vi "Autonomous Independent.vi"   [LabVIEW 2015]
doc: "This VI is called when autonomous begins, and will automatically be terminated when autonomous ends. You can carry out timed or sensor driven robot movement independently without needing to return to the caller."
uses:
  <vilib>/Rock Robotics/WPI/Solenoid/WPI_SolenoidValue.ctl
  <vilib>/Rock Robotics/WPI/Utilities/WPI_GetSetVariantRefNum.vi
  <vilib>/Rock Robotics/Network Tables/NT Read String.vi
  <vilib>/Rock Robotics/WPI/Solenoid/WPI_SolenoidSetEnum.vi
panel:
  # "Be sure to right-click and choose Data Operations>>Make Current Value default if you want to save the array values with the VI"
types:
  T1 = typedef "WPI_RobotDriveDevRef.ctl" = cluster{"DevStatus":errorcluster, "Motors[]":T2[], "Square Inputs":bool, "Max Output":dbl}
  T2 = typedef "WPI_MotorControlDeviceRef.ctl" = cluster{"DeviceStatus":errorcluster, "Type":T3, "PWM":cluster{"PWM Channel":T4, "DeadBand":T5}, "CAN":cluster{"Device Number":u8, "Control Mode":T6, "Semaphore":T7, "Max Vout":dbl, "TalonSRX Control Mode":T8}, "Invert":bool}
  T3 = typedef "WPI_MotorControlType.ctl" = enum16{"PWM", "CAN", "CANTalonSRX"}
  T4 = typedef "FPGA_DIOPWMChannel.ctl" = enum8{"PWM 0", "PWM 1", "PWM 2", "PWM 3", "PWM 4", "PWM 5", "PWM 6", "PWM 7", "PWM 8", "PWM 9", "PWM MXP 0", "PWM MXP 1", "PWM MXP 2", "PWM MXP 3", "PWM MXP 4", "PWM MXP 5", "PWM MXP 6", "PWM MXP 7", "PWM MXP 8", "PWM MXP 9", "Invalid"}
  T5 = typedef "WPI_PWMDeadband.ctl" = cluster{"Name":string, "maxPositivePwm":i32, "minPositivePwm":i32, "centerPwm":i32, "maxNegativePwm":i32, "minNegativePwm":i32, "angularRange":u16}
  T6 = typedef "WPI_CANJaguar_ControlMode.ctl" = enum8{"Percent VBus", "Current", "Speed", "Position", "Voltage"}
  T7 = typedef "Semaphore RefNum" = refnum<k1>
  T8 = typedef "WPI_CANTalonSRX_APIControlMode.ctl" = enum8{"Percent VBus", "Speed", "Position", "Slave", "Unchanged / Invalid", "Voltage Compensation", "Current", "Motion Profile"}
  T9 = typedef "WPI_SolenoidValue.ctl" = enum16{"Off", "On", "Forward", "Reverse"}
  T10 = typedef "WPI_SolenoidDevRef.ctl" = cluster{"DevStatus":errorcluster, "Pneumatics Control Module":u8, "Forward Solenoid Channel":T11, "Reverse Solenoid Channel":T11}
  T11 = typedef "WPI_SolenoidChannel.ctl" = enum8{"Solenoid 0", "Solenoid 1", "Solenoid 2", "Solenoid 3", "Solenoid 4", "Solenoid 5", "Solenoid 6", "Solenoid 7", "Invalid"}
  T12 = typedef "WPI_AccelerometerDevRef.ctl" = cluster{"DevStatus":errorcluster, "Scaling":T13, "Analog Channels":T14, "I2C Bus":T16, "SPI Bus":T17, "Accel Range":T18, "ADXL Axes":T19, "Handle":i32, "Device Address":u8, "Accel Type":enum16{"Analog", "ADXL345 I2C", "ADXL345 SPI", "Internal", "ADXL362 SPI"}}
  T13 = typedef "WPI_AccelerometerScaling.ctl" = cluster{"Gain (VoltsPerG)":dbl, "Center Voltage":dbl}
  T14 = typedef "WPI_AccelerometerAnalogChannels.ctl" = cluster{"X-Axis":T15, "Y-Axis":T15, "Z-Axis":T15}
  T15 = typedef "FPGA_AIChannel.ctl" = enum8{"AI 0", "AI 1", "AI 2", "AI 3", "AI MXP 0", "AI MXP 1", "AI MXP 2", "AI MXP 3", "Invalid"}
  T16 = typedef "i2c_bus.ctl" = enum16{"I2C On-Board", "I2C MXP", "Invalid"}
  T17 = typedef "spi_bus.ctl" = enum16{"SPI On-Board, CS0", "SPI On-Board, CS1", "SPI On-Board, CS2", "SPI On-Board, CS3", "SPI MXP", "Invalid"}
  T18 = typedef "ADXL345 Range.ctl" = u8
  T19 = typedef "WPI_AccelerometerADXL345 Axes.ctl" = cluster{"X-Axis":bool, "Y-Axis":bool, "Z-Axis":bool}
  T20 = cluster{"X-Axis":dbl, "Y-Axis":dbl, "Z-Axis":dbl}
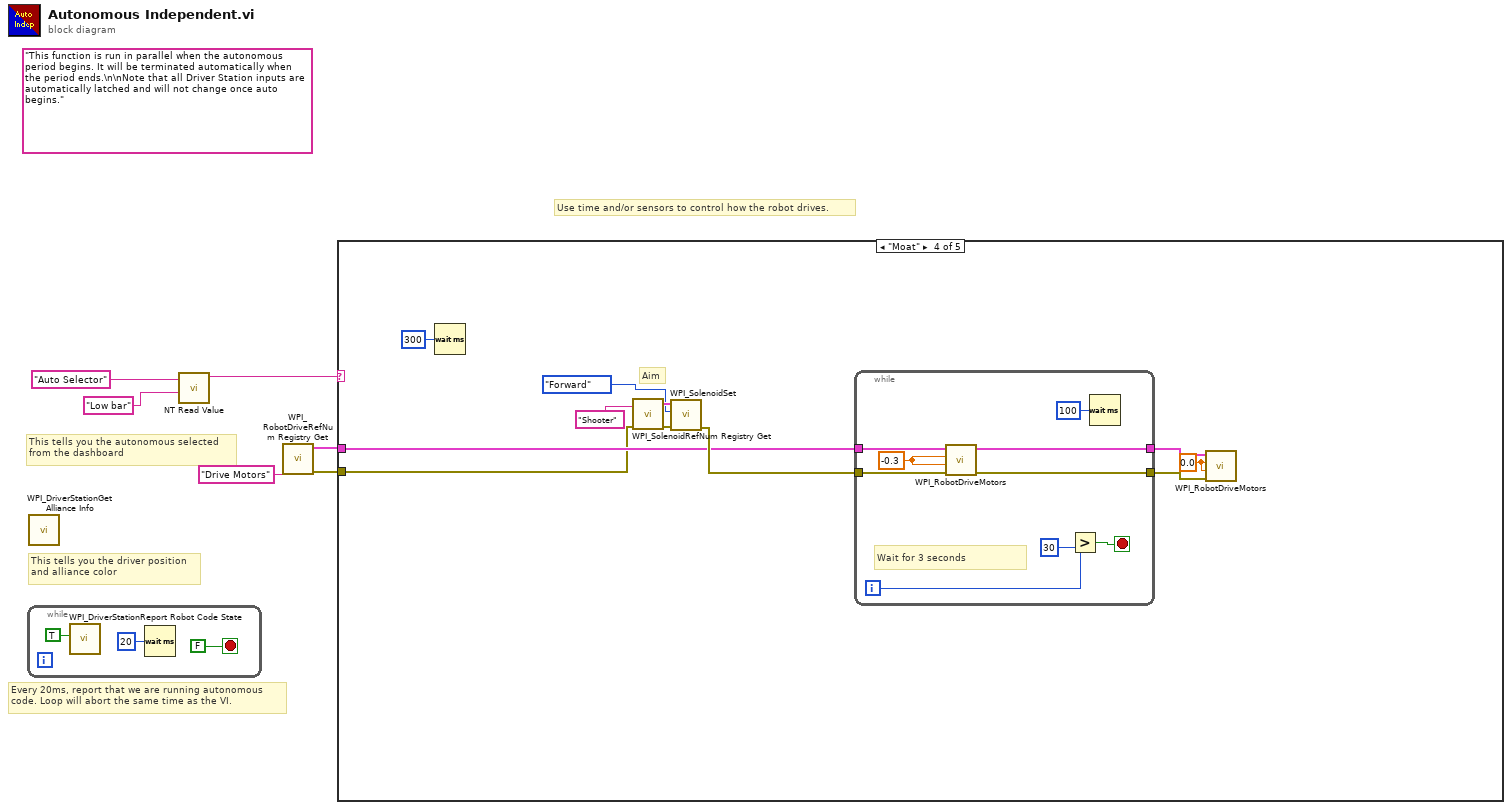
[diagram p0: block diagram]
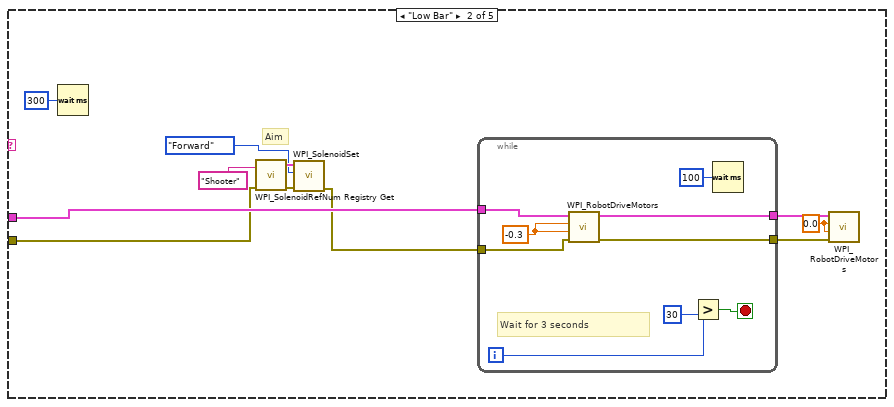
[diagram p3: hidden frame]
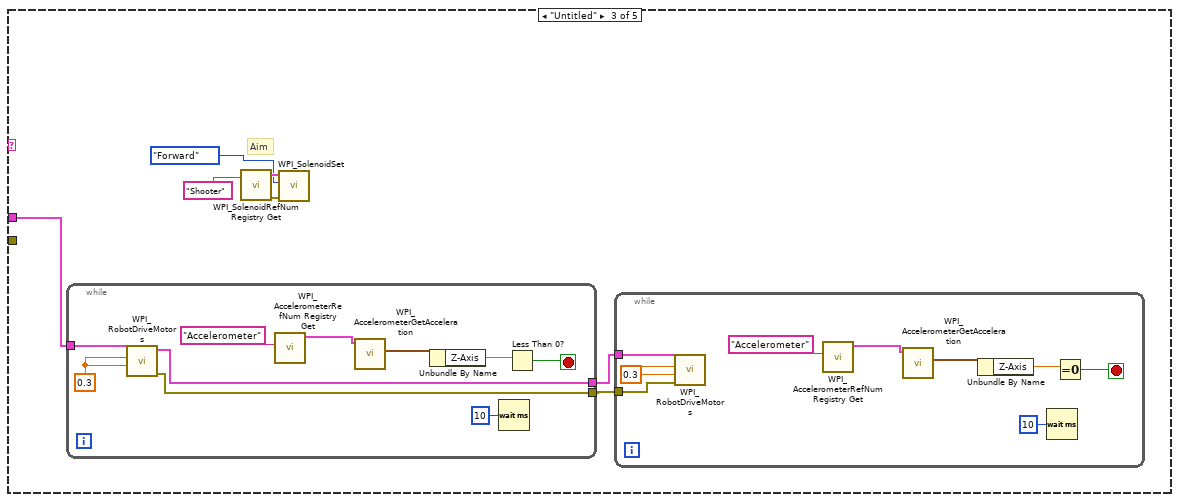
[diagram p4: hidden frame]
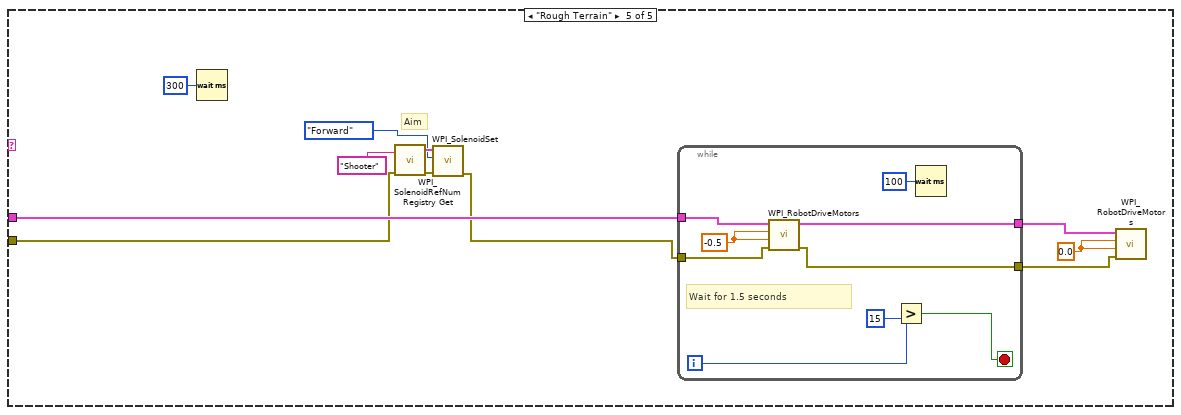
[diagram p5: hidden frame]
diagram:
  (unwired) "This function is run in parallel when the autonomous period begins. It will be terminated automatically when the period ends.\n\nNote that all Driver Station inputs are automatically latched and will not change once auto begins."
  # "This tells you the autonomous selected\nfrom the dashboard"
  # "Every 20ms, report that we are running autonomous\ncode. Loop will abort the same time as the VI."
  # "Use time and/or sensors to control how the robot drives."
  # "This tells you the driver position\nand alliance color"
  n1 = while {
    stop <- FALSE stop-if-true
    n2 = call <vilib>:"WPI_DriverStationReport Robot Code State.vi"("Autonomous"=TRUE) -> ()  [unwired: 10 in, 1 out]
    n3 = Wait (ms)(milliseconds to wait=u32 20) -> ()  [unwired: 1 out]
  }
  n4 = call <vilib>:"WPI_DriverStationGet Alliance Info.vi"() -> ()  [unwired: 12 out]
  n5 = call-poly <vilib>:"NT Read Value.vi"("Default Value"="Low bar", "Name"="Auto Selector") -> ("String"=w5:string)  [unwired: 8 in, 1 out]
  n6 = call <vilib>:"WPI_RobotDriveRefNum Registry Get.vi"("refnum name"="Drive Motors") -> ("error out"=w1:errorcluster, "RobotDriveDevRef"=w4:T1)  [unwired: 9 in]
  n7 = case shown="\"Moat\"" w5 {
    tunnel: w4 -> [_ w20 w34 w58 w86]
    tunnel: w1 -> [_ w14 _ w57 w77]
    frame Default {
      # "You can put your main auto here, or you can right-click on the case and make any\nother frame be the default case."
      # "This is the frame that will execute if no selection is made, or if it is not recognized"
    }
    frame "Low Bar" {
      w10 = 0.0 ("LeftSpeed")
      # "Aim"
      n8 = Wait (ms)(milliseconds to wait=u32 300) -> ()  [unwired: 1 out]
      n9 = call <vilib>:"WPI_SolenoidRefNum Registry Get.vi"("error in (no error)"=w14, "refnum name"="Shooter") -> ("error out"=w18:errorcluster, "SolenoidDevRef"=w19:T10)  [unwired: 8 in]
      n10 = call-poly <vilib>:"WPI_SolenoidSet.vi"("error in (no error)"=w18, "Value"=WPI_SolenoidValue."Forward", "SolenoidDevRef"=w19) -> ("error out"=w13:errorcluster)  [unwired: 7 in, 1 out]
      n11 = while {
        tunnel: w20 -> [w29]
        tunnel: w13 -> [w23]
        tunnel: [w22] -> w12
        tunnel: [w21] -> w11
        i -> [w26]
        stop <- w24 stop-if-true
        w28 = -0.3 ("LeftSpeed")
        # "Wait for 3 seconds"
        n12 = call <vilib>:"WPI_RobotDriveMotors.vi"("error in (no error)"=w23, "RightSpeed"=w28, "LeftSpeed"=w28, "RobotDriveDevRef"=w29) -> ("error out"=w21:errorcluster, "RobotDriveDevRef"=w22:T1)  [unwired: 5 in, 1 out]
        n13 = Greater?(x=w26, y=30) -> (0:w24:bool)
        n14 = Wait (ms)(milliseconds to wait=u32 100) -> ()  [unwired: 1 out]
      }
      n15 = call <vilib>:"WPI_RobotDriveMotors.vi"("error in (no error)"=w11, "RightSpeed"=w10, "LeftSpeed"=w10, "RobotDriveDevRef"=w12) -> ()  [unwired: 5 in, 3 out]
    }
    frame "Untitled" {
      # "Aim"
      n16 = while {
        tunnel: w34 -> [w55]
        tunnel: [w47] -> w36
        tunnel: [w46] -> w35
        stop <- w49 stop-if-true
        w54 = 0.3 ("LeftSpeed")
        n17 = call <vilib>:"WPI_RobotDriveMotors.vi"("RightSpeed"=w54, "LeftSpeed"=w54, "RobotDriveDevRef"=w55) -> ("error out"=w46:errorcluster, "RobotDriveDevRef"=w47:T1)  [unwired: 6 in, 1 out]
        n18 = call <vilib>:"WPI_AccelerometerRefNum Registry Get.vi"("refnum name"="Accelerometer") -> ("AccelerometerDevRef"=w52:T12)  [unwired: 9 in, 1 out]
        n19 = call <vilib>:"WPI_AccelerometerGetAcceleration.vi"("AccelerometerDevRef"=w52) -> ("Accelerations"=w51:T20)  [unwired: 8 in, 2 out]
        n20 = Unbundle By Name(w51) -> ("Z-Axis"=w50:dbl)
        n21 = Wait (ms)(milliseconds to wait=u32 10) -> ()  [unwired: 1 out]
        n22 = Less Than 0?(x=w50) -> (x < 0?=w49:bool)
      }
      n23 = call <vilib>:"WPI_SolenoidRefNum Registry Get.vi"("refnum name"="Shooter") -> ("error out"=w32:errorcluster, "SolenoidDevRef"=w33:T10)  [unwired: 9 in]
      n24 = call-poly <vilib>:"WPI_SolenoidSet.vi"("error in (no error)"=w32, "Value"=WPI_SolenoidValue."Forward", "SolenoidDevRef"=w33) -> ()  [unwired: 7 in, 2 out]
      n25 = while {
        tunnel: w36 -> [w45]
        tunnel: w35 -> [w37]
        stop <- w39 stop-if-true
        w44 = 0.3 ("LeftSpeed")
        n26 = call <vilib>:"WPI_RobotDriveMotors.vi"("error in (no error)"=w37, "RightSpeed"=w44, "LeftSpeed"=w44, "RobotDriveDevRef"=w45) -> ()  [unwired: 5 in, 3 out]
        n27 = call <vilib>:"WPI_AccelerometerRefNum Registry Get.vi"("refnum name"="Accelerometer") -> ("AccelerometerDevRef"=w42:T12)  [unwired: 9 in, 1 out]
        n28 = call <vilib>:"WPI_AccelerometerGetAcceleration.vi"("AccelerometerDevRef"=w42) -> ("Accelerations"=w41:T20)  [unwired: 8 in, 2 out]
        n29 = Unbundle By Name(w41) -> ("Z-Axis"=w40:dbl)
        n30 = Wait (ms)(milliseconds to wait=u32 10) -> ()  [unwired: 1 out]
        n31 = Equal To 0?(x=w40) -> (x = 0?=w39:bool)
      }
    }
    frame "Moat" {
      w59 = 0.0 ("LeftSpeed")
      # "Aim"
      n32 = Wait (ms)(milliseconds to wait=u32 300) -> ()  [unwired: 1 out]
      n33 = call <vilib>:"WPI_SolenoidRefNum Registry Get.vi"("error in (no error)"=w57, "refnum name"="Shooter") -> ("error out"=w65:errorcluster, "SolenoidDevRef"=w66:T10)  [unwired: 8 in]
      n34 = call-poly <vilib>:"WPI_SolenoidSet.vi"("error in (no error)"=w65, "Value"=WPI_SolenoidValue."Forward", "SolenoidDevRef"=w66) -> ("error out"=w62:errorcluster)  [unwired: 7 in, 1 out]
      n35 = while {
        tunnel: w58 -> [w75]
        tunnel: w62 -> [w69]
        tunnel: [w68] -> w61
        tunnel: [w67] -> w60
        i -> [w72]
        stop <- w70 stop-if-true
        w74 = -0.3 ("LeftSpeed")
        # "Wait for 3 seconds"
        n36 = call <vilib>:"WPI_RobotDriveMotors.vi"("error in (no error)"=w69, "RightSpeed"=w74, "LeftSpeed"=w74, "RobotDriveDevRef"=w75) -> ("error out"=w67:errorcluster, "RobotDriveDevRef"=w68:T1)  [unwired: 5 in, 1 out]
        n37 = Greater?(x=w72, y=30) -> (0:w70:bool)
        n38 = Wait (ms)(milliseconds to wait=u32 100) -> ()  [unwired: 1 out]
      }
      n39 = call <vilib>:"WPI_RobotDriveMotors.vi"("error in (no error)"=w60, "RightSpeed"=w59, "LeftSpeed"=w59, "RobotDriveDevRef"=w61) -> ()  [unwired: 5 in, 3 out]
    }
    frame "Rough Terrain" {
      w85 = 0.0 ("LeftSpeed")
      # "Aim"
      n40 = Wait (ms)(milliseconds to wait=u32 300) -> ()  [unwired: 1 out]
      n41 = call <vilib>:"WPI_SolenoidRefNum Registry Get.vi"("error in (no error)"=w77, "refnum name"="Shooter") -> ("error out"=w81:errorcluster, "SolenoidDevRef"=w82:T10)  [unwired: 8 in]
      n42 = call-poly <vilib>:"WPI_SolenoidSet.vi"("error in (no error)"=w81, "Value"=WPI_SolenoidValue."Forward", "SolenoidDevRef"=w82) -> ("error out"=w76:errorcluster)  [unwired: 7 in, 1 out]
      n43 = while {
        tunnel: w86 -> [w95]
        tunnel: w76 -> [w89]
        tunnel: [w88] -> w84
        tunnel: [w87] -> w83
        i -> [w92]
        stop <- w90 stop-if-true
        w94 = -0.5 ("LeftSpeed")
        # "Wait for 1.5 seconds"
        n44 = call <vilib>:"WPI_RobotDriveMotors.vi"("error in (no error)"=w89, "RightSpeed"=w94, "LeftSpeed"=w94, "RobotDriveDevRef"=w95) -> ("error out"=w87:errorcluster, "RobotDriveDevRef"=w88:T1)  [unwired: 5 in, 1 out]
        n45 = Greater?(x=w92, y=15) -> (0:w90:bool)
        n46 = Wait (ms)(milliseconds to wait=u32 100) -> ()  [unwired: 1 out]
      }
      n47 = call <vilib>:"WPI_RobotDriveMotors.vi"("error in (no error)"=w83, "RightSpeed"=w85, "LeftSpeed"=w85, "RobotDriveDevRef"=w84) -> ()  [unwired: 5 in, 3 out]
    }
  }
